vi "Auto_calibrate.vi"(3 "Mode":T4, 5 "Traverse line":T5 {"Row Duration (mins)" format="%#.1f"; "Row No" min=0; "Trace Gas Concentration (%)" min=0.0 format="%#.2f"; "Emission Rate (l/min)" format="%#.2f"; "Tunnel Speed" format="%#.2f"; "Start X" format="%#.2f"; "Start Y" format="%#.2f"; "Start Z" format="%#.2f"; "End X" format="%#.2f"; "End Y" format="%#.2f"; "End Z" format="%#.2f"; "Averaging time (min)" min=0.0 format="%#.1f"}) -> (0 "Error Messages":string, 1 "Status":T2, 2 "Traverse Out":T5 {"Row Duration (mins)" format="%#.1f"; "Row No" min=0; "Trace Gas Concentration (%)" min=0.0 format="%#.2f"; "Emission Rate (l/min)" format="%#.2f"; "Tunnel Speed" format="%#.2f"; "Start X" format="%#.2f"; "Start Y" format="%#.2f"; "Start Z" format="%#.2f"; "End X" format="%#.2f"; "End Y" format="%#.2f"; "End Z" format="%#.2f"; "Averaging time (min)" min=0.0 format="%#.1f"})   [LabVIEW 2010]
uses:
  Gen Trav/Traverse_cluster.ctl
  Gen Trav/Spacing.ctl
  Controls/Multi_run_mode.ctl
  Controls/User_Specific_mode.ctl
  Controls/Auto_Calib_Type.ctl
  Gen Trav/Multi_Run_Status.ctl
  Controls/Auto_Calib_Case.ctl
  Calibration/Calib_mode.ctl
  Controls/Save_Data.ctl
  Controls/Post_Process.ctl
  Controls/Setup.ctl
  Controls/App_Global.ctl
  Globals/Constants_global.vi
  Globals/Meas_global.vi
  Globals/Calib_global.vi
  Globals/Trav_pos_global.vi
  Globals/Plug_in_data_global.vi
  Globals/Extra_Commands_Global.vi
  <vilib>/Analysis/NI_AALBase.lvlib
panel:
  out "Minimum St Dev":dbl[](array[numeric])
  out "Time FFID valve moved":dbl
  out "Wait factor":dbl
  out "Establishment time":string
  out "Orig Calib file string":string
  out "Concentrations":dbl[](array[numeric])
  out "FFID St Dev":dbl[][](array[numeric]) format="%.2f"
  in  "Clear Calib History":bool
  out "Coefficients":dbl[][](array[numeric]) format="%.2f"
  out "Currently in Case":T1
  out "Valve position":dbl format="%.2f"
  out "Currently On":i32
  out "Values":dbl[][](array[numeric]) format="%.2f"
  out "FF Indexes":i16[](array[numeric])
  out "Ch No's":i16[](array[numeric])
  out "No of Calib Points":i32
  out "Root Name":string[](array[string])
  out "Original Calib File":path
  out "Calibration varying":T3
  in  "stop":bool
  out "New Calib Filenames":path[](array[path])
  # "Specific Argument Options\n      Tunnel Speed;1;2;3;4\nOR  Traverse Position\nOR   Concentration"
  # "X           Y            Z"
  # "Start"
  # "End"
  # "X           Y            Z"
  # "Start"
  # "End"
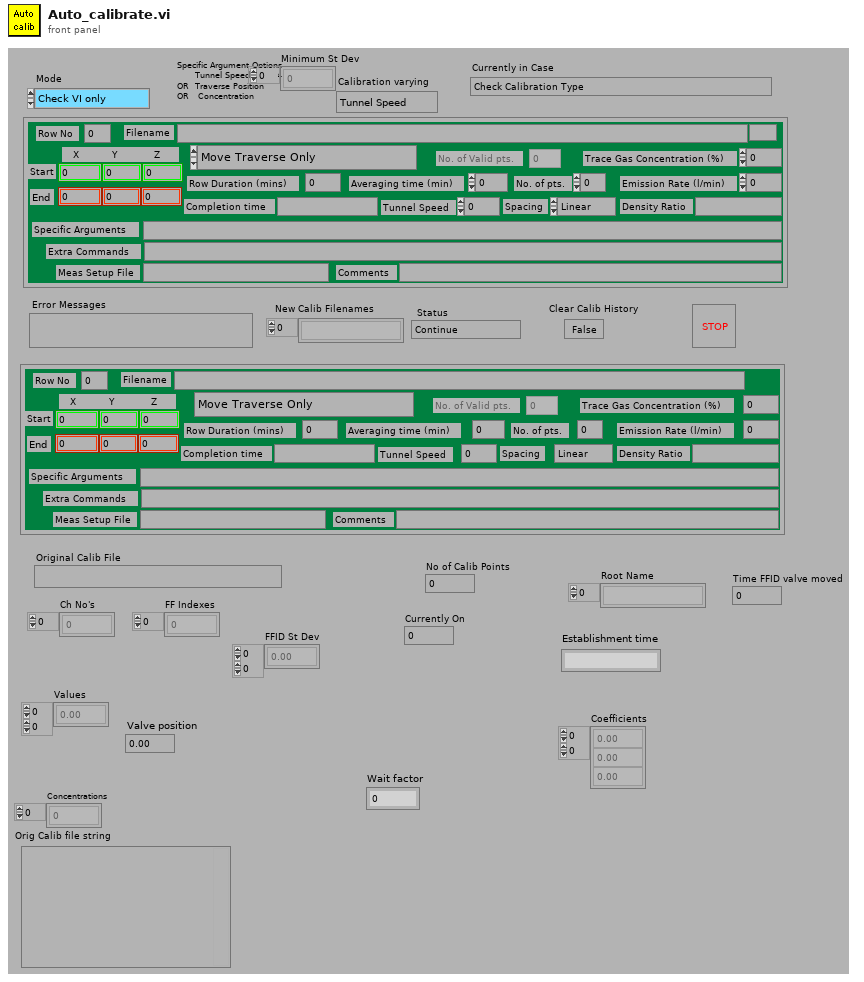
[diagram p1: front panel]
types:
  T1 = typedef "Auto_Calib_Case.ctl" = enum16{"Check Calibration Type", "Check if Original Calib file is Valid", "Get sampling rate etc. from meas setup file", "Setup Calibration Program", "Get Channel Numbers", "Check use latest selected on Mesurement setup files", "Create New Calib Filenames", "Setup Calibration Values in 2D array", "Create Measurement Setup File (Concentration Only)", "Are There Enough Calibration Points", "Set Measurement Conditions", "Measure Calibration Point", "Do Another Calibration Point?", "Skip Next Frame?", "Insert New calibration Filenames into Measurement Setup file", "Warn if FFID calibration is very non linear", "Warn if FFID variance is high", "Insert Bkgnd Variance into calib file", "Warn if FFID voltages are too low", "Warn if Current Calibration fit is poor", "Warn if Calibration Coefficients have significantly altered", "End"}
  T2 = typedef "Multi_Run_Status.ctl" = enum16{"Continue", "Jump to Next Point", "Jump to Next Row", "Jump To Fall Back", "Terminate Run"}
  T3 = typedef "Auto_Calib_Type.ctl" = enum16{"Tunnel Speed", "Traverse Position", "Concentration"}
  T4 = typedef "User_Specific_mode.ctl" = enum16{"Check VI only", "Run VI"}
  T5 = typedef "Traverse_cluster.ctl" = cluster{"Start X":dbl, "Start Y":dbl, "Start Z":dbl, "End X":dbl, "End Y":dbl, "End Z":dbl, "No. of pts.":i32, "Spacing":T6, "Filename":path, "Tunnel Speed":dbl, "Averaging time (min)":dbl, "Extra Commands":string, "Specific Arguments":string, "Emission Rate (l/min)":dbl, "Trace Gas Concentration (%)":dbl, "Density Ratio":string, "Comments":string, "Row No":i32, "Row Type Selector":T7, "Completion time":string, "Row Duration (mins)":dbl, "No. of Valid pts.":i32, "Meas Setup File":string}
  T6 = typedef "Spacing.ctl" = enum16{"Linear", "Log", "Gauss", "Specified", "N/A"}
  T7 = typedef "Multi_run_mode.ctl" = enum16{"Move Traverse Only", "Set Tunnel Speed Only", "Set Source Only", "Set Measurement Conditions", "Single Measurement", "Vertical Profile", "Lateral Profile", "Longitudinal Profile", "Explore Volume", "Multi-Axis Profile", "Auto Calibrate", "Meas Fast FID Bkgnd", "Check Beam Power", "Scanning Valve Measurement", "Run VI Named:", "Set ADAM Ch", "Wait (minutes)", "Send Message", "Synchronize With:", "Fall Back to this Row", "Turn Off Row Repeating", "Blank Row"}
  T8 = typedef "Calib_mode.ctl" = enum16{"Show Setup", "Take a New Calibration Point", "Refit Curve", "Setup Front Panel"}
  T9 = typedef "Save_Data.ctl" = enum16{"Save No Data", "Save Data"}
  T10 = typedef "Post_Process.ctl" = enum16{"Take New Data", "Post Process Raw Data File"}
  T11 = typedef "Setup.ctl" = enum16{"Run Program", "Show Setup", "Save Current Setup", "Setup Front Panel"}
  T12 = typedef "App_Global.ctl" = enum16{"Read Global", "Write to Global", "Initialise Array"}
  T13 = typedef "Cal_Inst_type.ctl" = enum16{"Propeller anemometer", "Pressure Transducer", "Hot wire", "Cross wire velocity", "Cross wire angle", "Generic Linear", "Generic Polynomial", "Generic BackPoly", "Fast FID", "Thermocouple", "Cold wire", "Pulsed Wire"}
  T14 = typedef "Ref_Inst_type.ctl" = enum16{"Propellor anemometer", "Pressure Transducer", "Raw voltage", "Pitot-static tube", "Preston tube", "Generic Linear", "Generic Polynomial", "Thermocouple", "LDA", "Enter Value", "ADAM Channel"}
  T15 = cluster{"2nd Ref type":T14, "2nd inst present":bool}
  T16 = cluster{"high limit (10V)":sgl, "low limit (-10V)":sgl, "Ch No":i16, "Var name":string}[]
  T17 = cluster{"high limit (10V)":sgl, "low limit (-10V)":sgl, "Ch No":i16, "Var name":string}
  T18 = typedef "Inst_type.ctl" = enum16{"Propeller anemometer", "Raw voltage", "Pressure Transducer", "Pitot-static tube", "Preston tube", "Hot wire", "Cross wire 1", "Cross wire 2", "Generic Linear", "Generic Polynomial", "Generic BackPoly", "Fast FID", "Thermocouple", "Cold wire", "Pulsed Wire", "LDA Vel", "LDA Tran time", "LDA Arr time"}
  T19 = cluster{"high limit (10V)":sgl, "low limit (-10V)":sgl, "Ch No":i16, "Calib filename":path, "Inst type":T18, "Symbol":string, "Move channel":bool, "Use Latest":bool, "D":dbl, "Ch Name":string}[]
  T20 = typedef "Status_Cluster.ctl" = cluster{"Status":T2, "Error Type":string, "Error Description":string}
  T21 = typedef "Valco_valve_ph.ctl" = u16
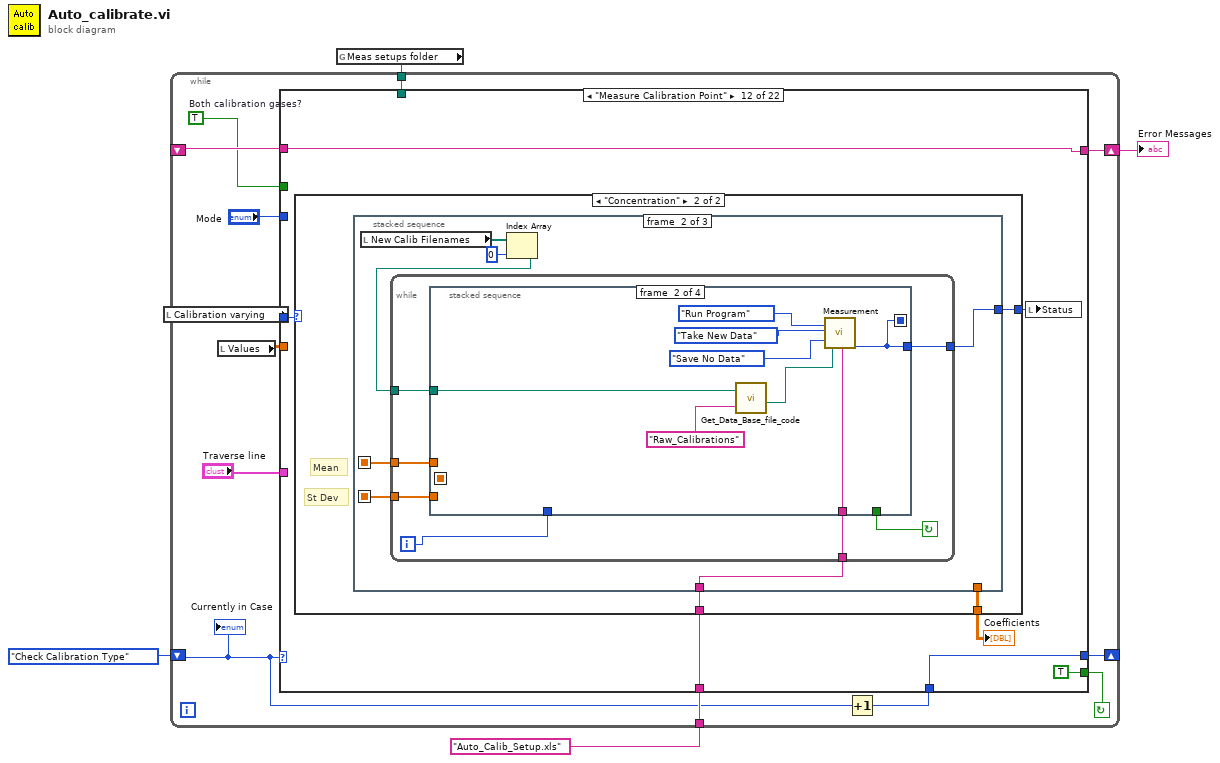
[diagram p0: block diagram]
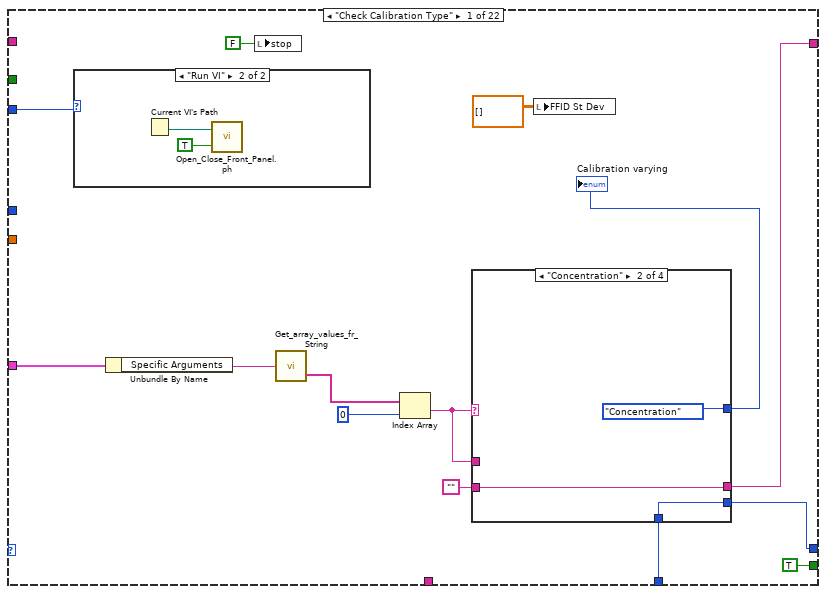
[diagram p2: hidden frame]
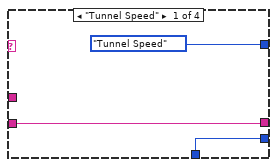
[diagram p4: hidden frame]
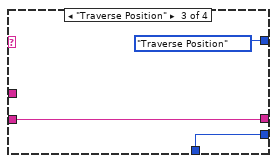
[diagram p5: hidden frame]
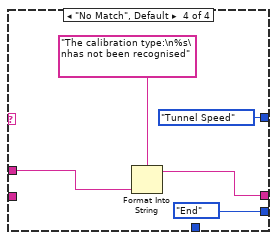
[diagram p6: hidden frame]
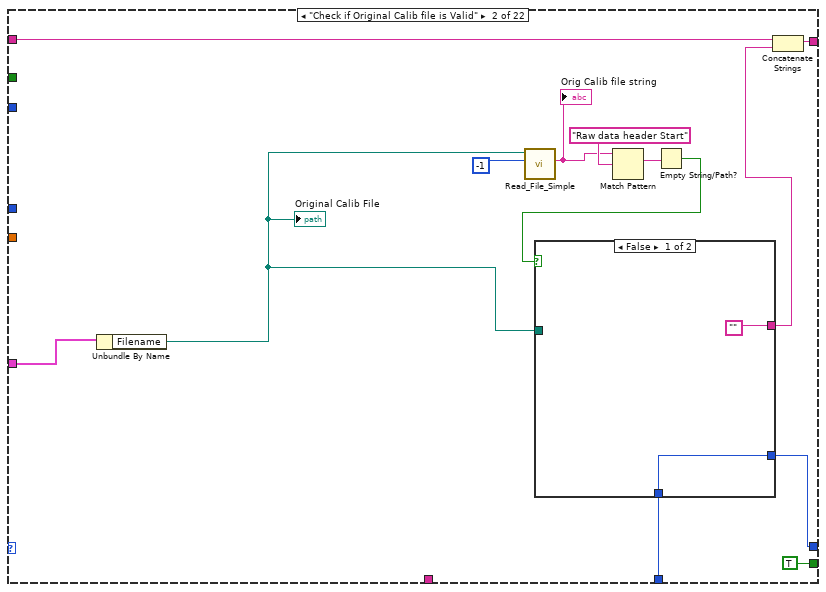
[diagram p7: hidden frame]
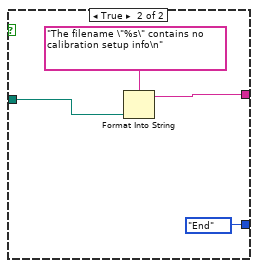
[diagram p8: hidden frame]
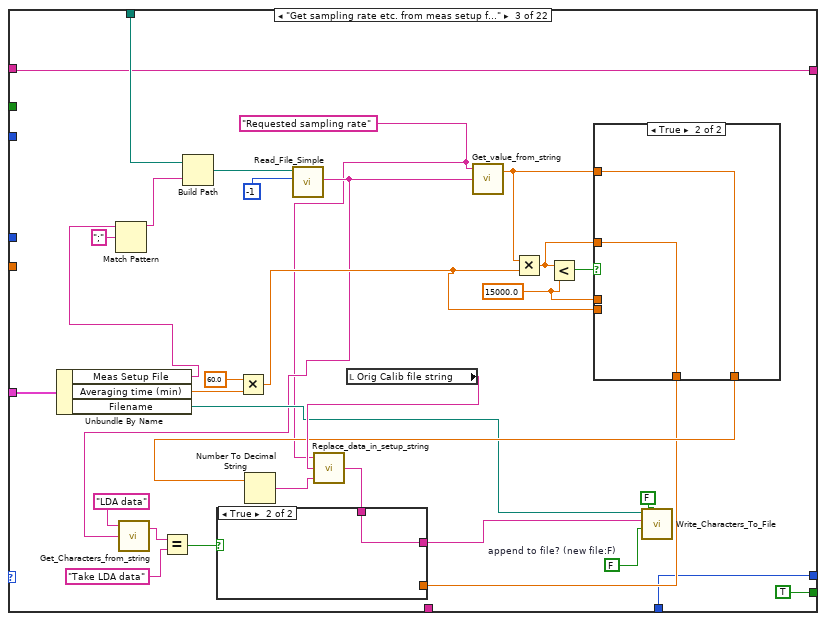
[diagram p9: hidden frame]
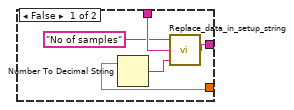
[diagram p10: hidden frame]
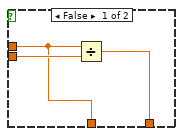
[diagram p11: hidden frame]
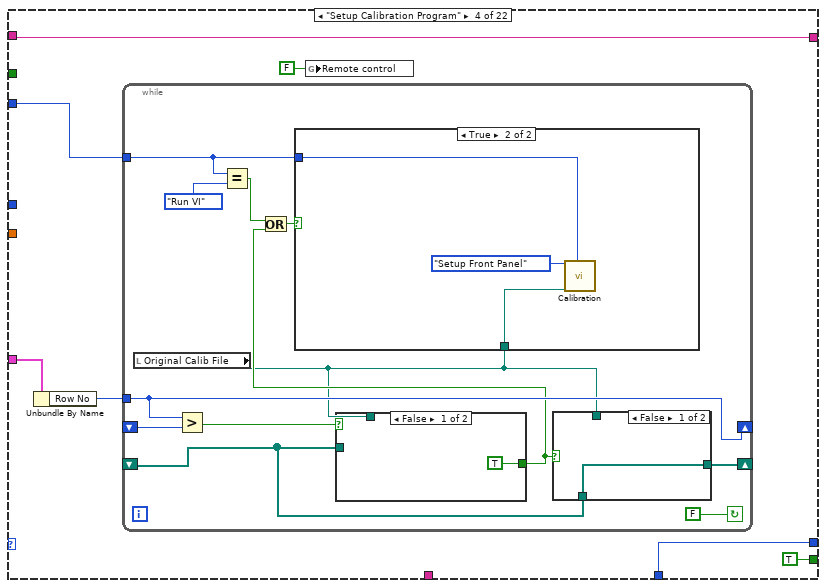
[diagram p12: hidden frame]
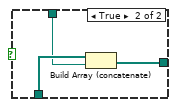
[diagram p13: hidden frame]
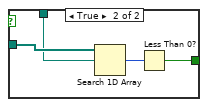
[diagram p15: hidden frame]
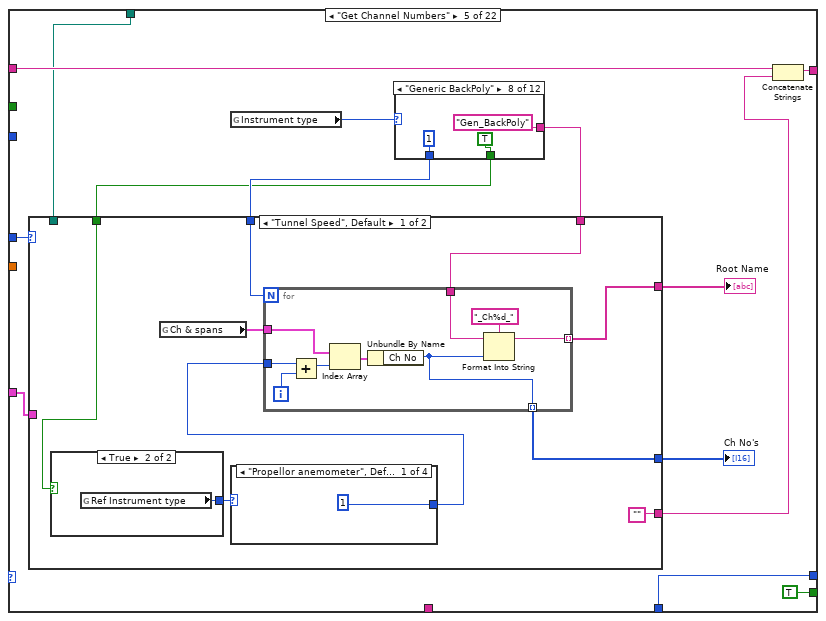
[diagram p16: hidden frame]
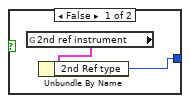
[diagram p17: hidden frame]
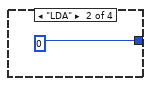
[diagram p18: hidden frame]
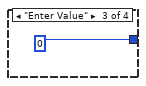
[diagram p19: hidden frame]
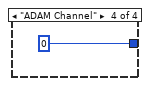
[diagram p20: hidden frame]
diagram:
  n1 = global read "Constants_global.vi" "Meas setups folder"() -> (w1:path)
  n2 = while {
    shift-left: _ -> [w9]
    shift-right: [w10] -> w3
    shift-left: Auto_Calib_Case."Check Calibration Type" ("Currently in Case") -> [w8]
    shift-right: [w7] -> _
    tunnel: "Auto_Calib_Setup.xls" -> [w17]
    tunnel: w1 -> [w5]
    stop <- w13 continue-if-true
    w6 = TRUE  # Both calibration gases?
    n3 = local read "Calibration varying"() -> (w12:T3)
    n4 = local read "Values"() -> (w11:dbl[][])
    n5 = Increment(x=w8) -> (x+1=w14:T1)
    n6 = case shown="\"Measure Calibration Point\"" w8 {
      tunnel: "Traverse line" -> [w31 w60 w98 w112 w143 _ _ w367 w400 _ w577 _ _ _ _ _ _ _ _ _ w993 w1024]
      tunnel: "Mode" -> [w22 _ _ w113 _ _ w318 _ w401 _ w572 _ w737 _ _ _ _ _ _ _ _ w1025]
      tunnel: w17 -> [_ _ _ _ _ _ _ _ w405 _ _ w649 _ _ _ _ _ _ _ _ _ _]
      tunnel: [w20 w50 w78 w115 w146 w264 w315 w358 w403 w540 w565 w648 w738 w764 w774 w795 w833 w898 w916 w972 w1016 w1030] -> w7
      tunnel: w14 -> [w21 w49 w78 w115 w146 w264 w315 w359 w403 w539 w559 w648 _ w763 w773 w795 w833 w898 w916 w972 w1016 w1030]
      tunnel: [TRUE TRUE TRUE TRUE TRUE TRUE TRUE TRUE w399 TRUE TRUE TRUE TRUE TRUE TRUE TRUE TRUE TRUE TRUE TRUE TRUE FALSE] -> w13
      tunnel: w12 -> [_ _ _ _ w150 _ w314 w365 _ _ w563 w650 w736 w762 w776 _ _ _ _ _ _ w1026]
      tunnel: w11 -> [_ _ _ _ _ _ _ _ w398 w549 w576 _ _ _ _ _ w840 _ w922 _ _ _]
      tunnel: [w24 w52 w76 w116 w147 w265 w329 w362 w404 w543 w560 w646 w735 w767 w780 w804 w847 w894 w923 w961 w1009 w1029] -> w10
      tunnel: w9 -> [_ w54 w76 w116 w149 w265 w329 w361 w404 w544 w560 w646 w735 w767 w780 w804 w847 w894 w923 w961 w1009 w1029]
      tunnel: w6 -> [_ _ _ _ _ _ _ w360 _ _ _ _ _ _ _ _ _ _ _ _ _ w1023]
      tunnel: w5 -> [_ _ w97 _ w142 w267 _ _ w402 _ _ _ _ _ _ _ _ _ _ _ _ _]
      frame "Check Calibration Type" {
        n7 = case shown="\"Run VI\"" w22 {
          frame "Check VI only" {
          }
          frame "Run VI" {
            n8 = Current VI's Path() -> (path=w32:path)
            n9 = call "Open_Close_Front_Panel.ph.vi"("Front Panel Window:Open"=TRUE, "VI path"=w32) -> ()  [unwired: 2 out]
          }
        }
        n10 = Unbundle By Name(w31) -> ("Specific Arguments"=w30:string)
        n11 = local write "stop"(FALSE) -> ()
        n12 = call "Get_array_values_fr_String.vi"("String Value"=w30) -> ("String array"=w29:string[])  [unwired: 1 out]
        n13 = Index Array(array=w29, index=0 ("Index")) -> (element=w27:string)
        n14 = case shown="\"Concentration\"" w27 {
          tunnel: [Auto_Calib_Type."Tunnel Speed" ("Calibration varying") Auto_Calib_Type."Concentration" ("Calibration varying") Auto_Calib_Type."Traverse Position" ("Calibration varying") Auto_Calib_Type."Tunnel Speed" ("Calibration varying")] -> w25
          tunnel: w27 -> [_ _ _ w46]
          tunnel: [w35 w38 w41 w44] -> w24
          tunnel: "" -> [w35 w38 w41 _]
          tunnel: w21 -> [w34 w37 w40 _]
          tunnel: [w34 w37 w40 Auto_Calib_Case."End" ("Currently in Case")] -> w20
          frame "Tunnel Speed" {
          }
          frame "Concentration" {
            (unwired) ""
          }
          frame "Traverse Position" {
          }
          frame "No Match", Default {
            n15 = Format Into String(format string="The calibration type:\n%s\nhas not been recognised" ("Format String"), w46) -> (resulting string=w44:string)  [unwired: 2 in, 1 out]
          }
        }
        "Calibration varying" <- w25
        n16 = local write "FFID St Dev"(dbl[][] [] ("FFID Variance")) -> ()
      }
      frame "Check if Original Calib file is Valid" {
        n17 = Unbundle By Name(w60) -> ("Filename"=w48:path)
        "Original Calib File" <- w48
        n18 = call "Read_File_Simple.vi"("Filename"=w48, "number of characters (all:-1)"=-1) -> ("string"=w57:string)  [unwired: 1 in, 7 out]
        "Orig Calib file string" <- w57
        n19 = Match Pattern(string=w57, regular expression="Raw data header Start") -> (match substring=w56:string)  [unwired: 4 out]
        n20 = Empty String/Path?(string/path=w56) -> (empty?=w55:bool)
        n21 = case shown="False" w55 {
          tunnel: w48 -> [_ w66]
          tunnel: ["" w64] -> w53
          tunnel: [w61 Auto_Calib_Case."End" ("Currently in Case")] -> w50
          tunnel: w49 -> [w61 _]
          frame False {
          }
          frame True {
            n22 = Format Into String(format string="The filename \"%s\" contains no calibration setup info\n" ("Format String"), w66) -> (resulting string=w64:string)  [unwired: 2 in, 1 out]
          }
        }
        n23 = Concatenate Strings(w54, w53) -> (w52:string)
      }
      frame "Get sampling rate etc. from meas setup file" {
        w79 = FALSE  # append to file? (new file:F)
        w67 = "Requested sampling rate"
        w86 = 15000.0 ("y")
        n24 = Unbundle By Name(w98) -> ("Meas Setup File"=w74:string, "Averaging time (min)"=w94:dbl, "Filename"=w81:path)
        n25 = Match Pattern(string=w74, regular expression=";") -> (before substring=w73:string)  [unwired: 4 out]
        n26 = Build Path(base path=w97, name or relative path=w73) -> (appended path=w95:path)
        n27 = Multiply(x=60.0, y=w94) -> (x*y=w85:dbl)
        n28 = call "Read_File_Simple.vi"("Filename"=w95, "number of characters (all:-1)"=-1) -> ("string"=w72:string)  [unwired: 1 in, 7 out]
        n29 = call "Get_Characters_from_string.vi"("Input string"=w72, "Variable name"="LDA data") -> ("Value"=w70:string)  [unwired: 1 in, 1 out]
        n30 = Equal?(x=w70, y="Take LDA data") -> (x = y?=w68:bool)
        n31 = local read "Orig Calib file string"() -> (w90:string)
        n32 = call "Get_value_from_string.vi"("Input string"=w72, "Variable name"=w67) -> ("Value"=w89:dbl)  [unwired: 1 in, 1 out]
        n33 = Multiply(x=w89, y=w85) -> (x*y=w84:dbl)
        n34 = Less?(x=w84, y=w86) -> (x < y?=w92:bool)
        n35 = case shown="True" w92 {
          tunnel: w89 -> [_ w109]
          tunnel: [w106 w109] -> w88
          tunnel: w86 -> [w105 _]
          tunnel: w85 -> [w107 _]
          tunnel: [w105 w108] -> w82
          tunnel: w84 -> [_ w108]
          frame False {
            n36 = Divide(x=w105, y=w107) -> (x/y=w106:dbl)
          }
          frame True {
          }
        }
        n37 = Number To Decimal String(number=w88) -> (decimal integer string=w87:string)  [unwired: 1 out]
        n38 = call "Replace_data_in_setup_string.vi"("New data string"=w87, "Input string"=w90, "Variable name"=w67) -> ("Appended string"=w83:string)
        n39 = case shown="True" w68 {
          tunnel: w83 -> [w103 w104]
          tunnel: w82 -> [w100 _]
          tunnel: [w99 w104] -> w80
          frame False {
            n40 = Number To Decimal String(number=w100) -> (decimal integer string=w101:string)  [unwired: 1 out]
            n41 = call "Replace_data_in_setup_string.vi"("New data string"=w101, "Input string"=w103, "Variable name"="No of samples") -> ("Appended string"=w99:string)
          }
          frame True {
          }
        }
        n42 = call "Write_Characters_To_File.vi"("file path (dialog if empty)"=w81, "advisory dialog? (display:T)"=FALSE, "character string"=w80, "append to file? (new file:F)"=w79) -> ()  [unwired: 1 in, 4 out]
      }
      frame "Setup Calibration Program" {
        n43 = Unbundle By Name(w112) -> ("Row No"=w111:i32)
        n44 = while {
          shift-left: _ -> [w120]
          shift-right: [w118] -> _
          tunnel: w111 -> [w127]
          shift-left: _ -> [w128]
          shift-right: [w127] -> _
          tunnel: w113 -> [w125]
          stop <- FALSE continue-if-true
          n45 = local read "Original Calib File"() -> (w119:path)
          n46 = Greater?(x=w127, y=w128) -> (0:w126:bool)
          n47 = Equal?(x=w125, y=User_Specific_mode."Run VI" ("Mode")) -> (x = y?=w123:bool)
          n48 = case shown="False" w126 {
            tunnel: w120 -> [_ w140]
            tunnel: w119 -> [_ w139]
            tunnel: [TRUE w137] -> w121
            frame False {
            }
            frame True {
              n49 = Search 1D Array(1D array=w140, element=w139) -> (index of element=w138:i32)  [unwired: 1 out]
              n50 = Less Than 0?(x=w138) -> (x < 0?=w137:bool)
            }
          }
          n51 = Or(x=w123, y=w121) -> (x .or. y?=w122:bool)
          n52 = case shown="True" w122 {
            tunnel: w125 -> [_ w135]
            tunnel: w119 -> [_ w134]
            frame False {
            }
            frame True {
              n53 = call "Calibration.vi"("Mode"=Calib_mode."Setup Front Panel", "Calib file"=w134, "Simulate/Run"=w135) -> ()  [unwired: 17 out]
            }
          }
          n54 = case shown="False" w121 {
            tunnel: w120 -> [w129 w132]
            tunnel: w119 -> [_ w131]
            tunnel: [w129 w130] -> w118
            frame False {
            }
            frame True {
              n55 = Build Array (concatenate)(w132, w131) -> (w130:path[])
            }
          }
        }
        n56 = global write "Meas_global.vi" "Remote control"(FALSE ("Remote control")) -> ()
      }
      frame "Get Channel Numbers" {
        n57 = global read "Calib_global.vi" "Instrument type"() -> (w154:T13)
        n58 = case shown="\"Generic BackPoly\"" w154 {
          tunnel: ["Prop" "Mano" "HW" "XW" "XW" "Gen_Lin" "Gen_Poly" "Gen_BackPoly" "FF" "Therm" "CW" "PWA"] -> w153
          tunnel: [1 1 1 2 2 1 1 1 1 1 1 1] -> w144
          tunnel: [TRUE TRUE TRUE TRUE FALSE TRUE TRUE TRUE TRUE TRUE TRUE TRUE] -> w141
          frame "Propeller anemometer" {
          }
          frame "Pressure Transducer" {
          }
          frame "Hot wire" {
          }
          frame "Cross wire velocity" {
          }
          frame "Cross wire angle" {
          }
          frame "Generic Linear" {
          }
          frame "Generic Polynomial" {
          }
          frame "Generic BackPoly" {
          }
          frame "Fast FID" {
          }
          frame "Thermocouple" {
          }
          frame "Cold wire" {
          }
          frame "Pulsed Wire" {
          }
        }
        n59 = case shown="\"Tunnel Speed\", Default" w150 {
          tunnel: w153 -> [w161 w197]
          tunnel: [w157 w196] -> w152
          tunnel: [w158 w194] -> w151
          tunnel: ["" w187] -> w148
          tunnel: w144 -> [w159 _]
          tunnel: w143 -> [_ w186]
          tunnel: w142 -> [_ w185]
          tunnel: w141 -> [w155 _]
          frame "Tunnel Speed", Default {
            n60 = case shown="True" w155 {
              tunnel: [w164 w166] -> w163
              frame False {
                n61 = global read "Calib_global.vi" "2nd ref instrument"() -> (w165:T15)
                n62 = Unbundle By Name(w165) -> ("2nd Ref type"=w164:T14)
              }
              frame True {
                n63 = global read "Calib_global.vi" "Ref Instrument type"() -> (w166:T14)
              }
            }
            n64 = global read "Calib_global.vi" "Ch & spans"() -> (w160:T16)
            n65 = case shown="\"Propellor anemometer\", Default" w163 {
              tunnel: [1 i16 0 0 0] -> w156
              frame "Propellor anemometer", Default {
              }
              frame "LDA" {
              }
              frame "Enter Value" {
              }
              frame "ADAM Channel" {
              }
            }
            n66 = for {
              N: w159 -> [_]
              tunnel: [w173] -> w158 mode=indexing
              tunnel: w161 -> [w172]
              tunnel: w160 -> [w171]
              tunnel: [w170] -> w157 mode=indexing
              tunnel: w156 -> [w168]
              i -> [w169]
              n67 = Add(x=w168, y=w169) -> (x+y=w167:i32)
              n68 = Index Array(array=w171, index=w167) -> (element=w175:T17)
              n69 = Unbundle By Name(w175) -> ("Ch No"=w173:i16)
              n70 = Format Into String(format string="_Ch%d_" ("Format String"), initial string=w172, w173) -> (resulting string=w170:string)  [unwired: 1 in, 1 out]
            }
          }
          frame "Concentration" {
            w193 = i16[] []
            n71 = Unbundle By Name(w186) -> ("Meas Setup File"=w181:string)
            n72 = Match Pattern(string=w181, regular expression=";") -> (before substring=w180:string)  [unwired: 4 out]
            n73 = Build Path(base path=w185, name or relative path=w180) -> (appended path=w184:path)
            n74 = call "Read_raw_inst_setup.vi"("Setup file"=w184) -> ("Ch & spans choices"=w183:T19)  [unwired: 18 out]
            n75 = for {
              tunnel: w183 -> [w208] mode=indexing
              tunnel: w197 -> [w207]
              shift-right: [w203] -> w196
              shift-left: string[] [] -> [w204]
              shift-right: [w201] -> w194
              shift-left: w193 -> [w202]
              shift-right: [w200] -> w192
              shift-left: w193 -> [w199]
              i -> [w198]
              n76 = Unbundle By Name(w208) -> ("Ch No"=w206:i16, "Inst type"=w205:T18)
              n77 = case shown="\"Fast FID\"" w205 {
                tunnel: w207 -> [_ w213]
                tunnel: w206 -> [_ w215]
                tunnel: w204 -> [w211 w223]
                tunnel: [w211 w222] -> w203
                tunnel: w202 -> [w210 w221]
                tunnel: [w210 w220] -> w201
                tunnel: w199 -> [w209 w218]
                tunnel: [w209 w219] -> w200
                tunnel: w198 -> [_ w217]
                frame "Generic Linear", Default {
                }
                frame "Fast FID" {
                  n78 = To Word Integer(number=w217) -> (16bit integer=w216:i16)
                  n79 = Format Into String(format string="_Ch%d_", initial string=w213, w215) -> (resulting string=w212:string)  [unwired: 1 in, 1 out]
                  n80 = Build Array (concatenate)(w221, w215) -> (w220:i16[])
                  n81 = Build Array (concatenate)(w218, w216) -> (w219:i16[])
                  n82 = Build Array (concatenate)(w223, w212) -> (w222:string[])
                }
              }
            }
            "FF Indexes" <- w192
            n83 = Array Size(array=w192) -> (size(s)=w191:i32)
            n84 = Greater Than 0?(x=w191) -> (x > 0?=w190:bool)
            n85 = Select(t="", s=w190, f="There are no Fast Fid channels selected on the current setup of the measurement program.") -> (s? t:f=w187:string)
          }
        }
        "Root Name" <- w152
        "Ch No's" <- w151
        n86 = Concatenate Strings(w149, w148) -> (w147:string)
      }
      frame "Check use latest selected on Mesurement setup files" {
        n87 = global read "Trav_pos_global.vi" "Measurement setup files"() -> (w260:string[])
        n88 = local read "Ch No's"() -> (w266:i16[])
        n89 = Build Array (concatenate)(w260, "Current_Setup.xls") -> (w261:string[])
        n90 = for {
          tunnel: w267 -> [w270]
          tunnel: w261 -> [w269] mode=indexing
          tunnel: w266 -> [w268]
          n91 = stacked-sequence {
            seq-local: [w271 _ _] -> [_ w277 w305]
            seq-local: [_ w275 _] -> [_ _ w303]
            tunnel: w270 -> [w274 _ w302]
            tunnel: w269 -> [w273 _ w301]
            tunnel: w268 -> [_ w276 _]
            frame #0 {
              n92 = Build Path(base path=w274, name or relative path=w273) -> (appended path=w272:path)
              n93 = call "Read_File_Simple.vi"("Filename"=w272) -> ("string"=w271:string)  [unwired: 2 in, 7 out]
            }
            frame #1 {
              n94 = while {
                shift-right: [w282] -> w275
                shift-left: w277 -> [w283]
                tunnel: w276 -> [w286]
                i -> [w290]
                stop <- w279 continue-if-true
                n95 = Increment(x=w290) -> (x+1=w284:i32)
                n96 = Format Into String(format string="An ch %d Ch No", w284) -> (resulting string=w289:string)  [unwired: 2 in, 1 out]
                n97 = call "Get_value_from_string.vi"("Input string"=w283, "Variable name"=w289) -> ("Status"=w288:enum16{"Char in string", "Char not in string"}, "Value"=w287:dbl)  [unwired: 1 in]
                n98 = To Long Integer(number=w287) -> (32bit integer=w285:i32)
                n99 = Search 1D Array(1D array=w286, element=w285) -> (index of element=w281:i32)  [unwired: 1 in]
                n100 = Greater Or Equal To 0?(x=w281) -> (x >= 0?=w280:bool)
                n101 = case shown="\"Char in string\"" w288 {
                  tunnel: [TRUE FALSE] -> w279
                  frame "Char in string" {
                  }
                  frame "Char not in string" {
                  }
                }
                n102 = And(x=w280, y=w279) -> (x .and. y?=w278:bool)
                n103 = case shown="True" w278 {
                  tunnel: w284 -> [w294 _]
                  tunnel: w283 -> [w293 w298]
                  tunnel: [w292 w298] -> w282
                  frame True {
                    n104 = Format Into String(format string="An ch %d Use latest Calib", w294) -> (resulting string=w296:string)  [unwired: 2 in, 1 out]
                    n105 = call "Replace_data_in_setup_string.vi"("New data string"="TRUE" ("Replace with"), "Input string"=w293, "Variable name"=w296) -> ("Appended string"=w292:string)
                  }
                  frame False {
                  }
                }
              }
            }
            frame #2 {
              n106 = Equal?(x=w305, y=w303) -> (x = y?=w304:bool)
              n107 = case shown="True" w304 {
                tunnel: w302 -> [w308 _]
                tunnel: w303 -> [w311 _]
                tunnel: w301 -> [w307 _]
                frame False {
                  w310 = FALSE  # append to file? (new file:F)
                  n108 = Build Path(base path=w308, name or relative path=w307) -> (appended path=w306:path)
                  n109 = call "Write_Characters_To_File.vi"("file path (dialog if empty)"=w306, "advisory dialog? (display:T)"=FALSE, "character string"=w311, "append to file? (new file:F)"=w310) -> ()  [unwired: 1 in, 4 out]
                }
                frame True {
                }
              }
            }
          }
        }
      }
      frame "Create New Calib Filenames" {
        n110 = local read "Original Calib File"() -> (w327:path)
        n111 = Get Date/Time String(date format (0)=enum16{"short", "long", "abbreviated"}."short") -> (date string=w322:string)  [unwired: 3 out]
        n112 = Strip Path(path=w327) -> (stripped path=w317:path)  [unwired: 1 out]
        n113 = local read "Root Name"() -> (w313:string[])
        n114 = case shown="\"Tunnel Speed\", Default" w314 {
          tunnel: w313 -> [_ w334]
          tunnel: [1 w333] -> w312
          frame "Tunnel Speed", Default {
          }
          frame "Concentration" {
            n115 = Array Size(array=w334) -> (size(s)=w333:i32)
          }
        }
        n116 = call "Replace_Character.vi"("Replace with"="-", "Input String"=w322, "Search For"="/") -> ("Output string"=w319:string)  [unwired: 1 out]
        n117 = List Folder(path=w317) -> (filenames=w331:string[])  [unwired: 1 in, 5 out]
        n118 = To Upper Case(1:w331) -> (0:w330:string[])
        n119 = for {
          N: w312 -> [_]
          tunnel: w313 -> [w337] mode=indexing
          tunnel: w330 -> [w341]
          tunnel: w317 -> [w340]
          tunnel: [w336] -> w326 mode=indexing
          tunnel: w319 -> [w338]
          tunnel: w318 -> [w335]
          n120 = while {
            tunnel: w337 -> [w348]
            tunnel: w338 -> [w349]
            tunnel: [w344] -> w339
            tunnel: w341 -> [w351]
            i -> [w353]
            stop <- w355 continue-if-true
            n121 = Increment(x=w353) -> (x+1=w350:i32)
            n122 = Format Into String(format string="%s_%d.xls" ("Format String"), initial string=w348, w349, w350) -> (resulting string=w345:string)  [unwired: 1 in, 1 out]
            n123 = call "Replace_Character.vi"("Replace with"="_", "Input String"=w345, "Search For"=" ") -> ("Output string"=w344:string)  [unwired: 1 out]
            n124 = To Upper Case(1:w344) -> (0:w354:string)
            n125 = Search 1D Array(1D array=w351, element=w354) -> (index of element=w356:i32)  [unwired: 1 out]
            n126 = Not Equal?(x=w356, y=-1) -> (x != y?=w355:bool)
          }
          n127 = Build Path(base path=w340, name or relative path=w339) -> (appended path=w336:path)
          n128 = case shown="\"Run VI\"" w335 {
            tunnel: w336 -> [_ w342]
            frame "Check VI only" {
            }
            frame "Run VI" {
              n129 = call "Calibration.vi"("Mode"=Calib_mode."Setup Front Panel", "Calib file"=w342) -> ()  [unwired: 1 in, 17 out]
            }
          }
        }
        "New Calib Filenames" <- w326
        n130 = Index Array(array=w326, index=0 ("Index")) -> (element=w324:path)
        n131 = global write "Meas_global.vi" "Results file"(w324) -> ()
        "Establishment time" <- "!Establish Exp Conditions (s) = 15" ("Message")
      }
      frame "Setup Calibration Values in 2D array" {
        n132 = case shown="\"Concentration\"" w365 {
          tunnel: [w376 w382 w397] -> w364
          tunnel: w367 -> [w371 _ w396]
          tunnel: ["" "" w395] -> w363
          tunnel: w360 -> [_ w380 _]
          tunnel: w359 -> [w370 w379 w394]
          tunnel: [w369 w379 w393] -> w358
          frame "Tunnel Speed" {
            n133 = Unbundle By Name(w371) -> ("Specific Arguments"=w374:string)
            n134 = call "Get_array_values_fr_String.vi"("String Value"=w374) -> ("Numeric Array"=w372:dbl[])  [unwired: 1 out]
            n135 = Array Subset(array=w372, index=1 ("Array Index")) -> (w368:dbl[])  [unwired: 1 in]
            n136 = for {
              tunnel: w368 -> [w378] mode=indexing
              tunnel: [w377] -> w376 mode=indexing
              n137 = Build Array(w378) -> (w377:dbl[])
            }
            n138 = Increment(x=w370) -> (x+1=w369:T1)
          }
          frame "Concentration" {
            n139 = case shown="True" w380 {
              tunnel: [w384 w388] -> w383
              frame True {
                n140 = Build Array(3.0, 2.0, 1.0) -> (w384:dbl[])
              }
              frame False {
                n141 = Build Array(1.0, 3.0) -> (w388:dbl[])
              }
            }
            n142 = for {
              tunnel: w383 -> [w392] mode=indexing
              tunnel: [w391] -> w382 mode=indexing
              n143 = Build Array(w392) -> (w391:dbl[])
            }
          }
          frame "Traverse Position" {
            n144 = call "Create_Pos_array.vi"("Traverse line"=w396) -> ("Error Messages"=w395:string, "Array of Positions"=w397:dbl[][])  [unwired: 5 in, 2 out]
            n145 = Increment(x=w394) -> (x+1=w393:T1)
          }
        }
        "Values" <- w364
        n146 = Concatenate Strings(w361, w363) -> (w362:string)
      }
      frame "Create Measurement Setup File (Concentration Only)" {
        n147 = stacked-sequence {
          seq-local: [w416 _ _ _ _ _ _] -> [_ w435 _ _ _ _ _]
          seq-local: [_ w433 _ _ _ _ _] -> [_ _ w456 _ _ _ _]
          seq-local: [_ _ _ _ w478 _ _] -> [_ _ _ _ _ w491 _]
          seq-local: [_ _ _ _ w483 _ _] -> [_ _ _ _ _ w492 _]
          tunnel: w402 -> [w407 _ w457 _ _ _ _]
          tunnel: w405 -> [_ _ w458 _ _ _ _]
          tunnel: w401 -> [_ _ _ w464 _ w494 w524]
          tunnel: w400 -> [w413 _ _ _ w490 w495 _]
          tunnel: [_ _ _ _ _ w493 _] -> w399
          tunnel: w398 -> [_ _ _ w467 _ _ _]
          frame #0 {
            w420 = TRUE  # Show Dialog?
            n148 = Unbundle By Name(w413) -> ("Meas Setup File"=w414:string)
            n149 = Match Pattern(string=w414, regular expression=";") -> (before substring=w412:string)  [unwired: 4 out]
            n150 = Build Path(base path=w407, name or relative path=w412) -> (appended path=w421:path)
            n151 = Format Into String(format string="Meas Setup File   %s", w407) -> (resulting string=w406:string)  [unwired: 2 in, 1 out]
            n152 = call "Read_spec_No_of_Characters.vi"("Filename"=w421) -> ("character string"=w422:string)  [unwired: 1 out]
            n153 = call "Get_string_subset.vi"("String Name"=w406, "Show Dialog?"=w420, "String to split"=w422, "File Label"="Raw data header") -> ("Output string"=w409:string)  [unwired: 1 out]
            n154 = call "Get_value_from_string.vi"("Input string"=w409, "Variable name"="No of analogue inst") -> ("Value"=w410:dbl)  [unwired: 1 in, 1 out]
            n155 = for {
              N: w410 -> [_]
              shift-right: [w424] -> w419
              shift-left: w409 -> [w426]
              i -> [w430]
              n156 = Increment(x=w430) -> (x+1=w429:i32)
              n157 = Number To Decimal String(number=w429) -> (decimal integer string=w432:string)  [unwired: 1 out]
              n158 = Concatenate Strings("An ch ", w432, " Inst type") -> (w427:string)
              n159 = call "Replace_data_in_setup_string.vi"("New data string"="Raw voltage", "Input string"=w426, "Variable name"=w427) -> ("Appended string"=w424:string)
            }
            n160 = call "Replace_data_in_setup_string.vi"("New data string"="No LDA data", "Input string"=w419, "Variable name"="LDA data" ("Label for characters")) -> ("Appended string"=w416:string)
          }
          frame #1 {
            n161 = global read "Calib_global.vi" "New Setup String"() -> (w436:string)
            n162 = for {
              N: 4 -> [_]
              shift-right: [w441] -> w433
              shift-left: w435 -> [w442]
              tunnel: w436 -> [w438]
              i -> [w440]
              n163 = case shown="3" w440 {
                tunnel: [w445 w448 w451 "No of blocks"] -> w439
                tunnel: w438 -> [w444 w447 w450 _]
                tunnel: [w443 w446 w449 "1" ("Value")] -> w437
                frame 0, Default {
                  w445 = "No of samples"
                  n164 = call "Get_Characters_from_string.vi"("Input string"=w444, "Variable name"=w445) -> ("Value"=w443:string)  [unwired: 1 in, 1 out]
                }
                frame 2 {
                  w448 = "Actual sampling rate"
                  n165 = call "Get_Characters_from_string.vi"("Input string"=w447, "Variable name"=w448) -> ("Value"=w446:string)  [unwired: 1 in, 1 out]
                }
                frame 3 {
                  w451 = "Board type"
                  n166 = call "Get_Characters_from_string.vi"("Input string"=w450, "Variable name"=w451) -> ("Value"=w449:string)  [unwired: 1 in, 1 out]
                }
                frame 1 {
                }
              }
              n167 = call "Replace_data_in_setup_string.vi"("New data string"=w437, "Input string"=w442, "Variable name"=w439) -> ("Appended string"=w441:string)
            }
          }
          frame #2 {
            w462 = FALSE  # advisory dialog? (display:T)
            w463 = FALSE  # append to file? (new file:F)
            n168 = call "Remove_Plug_Ins_etc.vi"("Input String"=w456) -> ("Output string"=w455:string)
            n169 = call "Add_label_to_string.vi"("String to write"=w455, "File Label"="Raw data header") -> ("Output string"=w459:string)
            n170 = Build Path(base path=w457, name or relative path=w458) -> (appended path=w454:path)
            n171 = call "Add_length_to_string.vi"("String in"=w459) -> ("String out"=w461:string)
            n172 = call "Write_Characters_To_File.vi"("file path (dialog if empty)"=w454, "advisory dialog? (display:T)"=w462, "character string"=w461, "append to file? (new file:F)"=w463) -> ()  [unwired: 1 in, 4 out]
          }
          frame #3 {
            w466 = 0 ("Index")
            w471 = 0.0 ("Input Element")
            n173 = Index Array(array=w467, index (row)=w466, index (col)=w466) -> (element=w465:dbl)
            n174 = case shown="\"Run VI\"" w464 {
              tunnel: w465 -> [_ w474]
              frame "Check VI only" {
              }
              frame "Run VI" {
                n175 = flat-sequence {
                  tunnel: w474 -> [w475]
                  frame #0 {
                    n176 = call "Fast_FID_Valve_Control.vi"("Requested Position"=w475) -> ()  [unwired: 7 out]
                  }
                  frame #1 {
                    n177 = Get Date/Time In Seconds() -> (seconds since 1Jan1904=w477:timestamp)
                    n178 = To Double Precision Float(number=w477) -> (double precision float=→"Time FFID valve moved":dbl)
                  }
                }
              }
            }
            n179 = Build Array("GMU:Calibration:Gas 1", "GMU:Calibration:Gas 2") -> (w473:string[])
            n180 = call "Get_Current_Scan_client.vi"("ADAM Ch Names"=w473) -> ("Numerical Values"=w472:dbl[])  [unwired: 3 out]
            n181 = Build Array (concatenate)(w471, w471, w472, w471) -> (→"Concentrations":dbl[])
          }
          frame #4 {
            n182 = Unbundle By Name(w490) -> ("Extra Commands"=w489:string, "Start X"=w487:dbl, "Start Y"=w486:dbl, "Start Z"=w485:dbl)
            n183 = Build Array(w487, w486, w485) -> (w483:dbl[])
            n184 = call "Which_Trav_Setup.vi"("Extra Command String"=w489) -> ("Traverse Setup"=w488:string)
            n185 = call "Read_Traverse_Pos_File.vi"("Traverse Name"=w488) -> ("Tunnel Coordinates"=w484:dbl[])
            n186 = Subtract(x=w484, y=w483) -> (x-y=w482:dbl[])
            n187 = Absolute Value(x=w482) -> (abs(x)=w481:dbl[])
            n188 = Less?(x=w481, y=0.5) -> (x < y?=w479:bool[])
            n189 = And Array Elements(Boolean array=w479) -> (logical AND=w478:bool)
          }
          frame #5 {
            n190 = case shown="False" w491 {
              tunnel: w495 -> [w505 _]
              tunnel: w494 -> [w501 _]
              tunnel: [w497 TRUE] -> w493
              tunnel: w492 -> [w496 _]
              frame False {
                w500 = dbl[] [30.0, 15.0, 0.0] ("appended array")
                n191 = call "Coordinate_Trans_.vi"("Input Position"=w496) -> ("X"=w502:dbl, "Y"=w503:dbl, "Z"=w504:dbl)
                n192 = Array Size(array=w500) -> (size(s)=w499:i32)
                n193 = Decrement(x=w499) -> (x-1=w498:i32)
                n194 = while {
                  tunnel: w501 -> [w514]
                  tunnel: w505 -> [w520]
                  tunnel: w500 -> [w519] mode=indexing
                  tunnel: w504 -> [w517]
                  tunnel: w503 -> [w516]
                  tunnel: w502 -> [w515]
                  tunnel: w498 -> [w510]
                  tunnel: [w506] -> w497
                  i -> [w511]
                  stop <- w507 continue-if-true
                  n195 = Add(x=w517, y=w519) -> (x+y=w518:dbl)
                  n196 = Less?(x=w511, y=w510) -> (x < y?=w508:bool)
                  n197 = Bundle By Name(cluster=w520, "Start X"=w515, "Start Y"=w516, "Start Z"=w518) -> (w521:T5)
                  n198 = call "Set_Traverse_Position.vi"("Simulate/Run"=w514, "Currently on Point"=1, "Traverse line"=w521) -> ("Status Cluster"=w509:T20)  [unwired: 2 out]
                  n199 = Unbundle By Name(w509) -> ("Status"=w512:T2)
                  n200 = call "Prog_Status_Handler.vi"("Status Cluster"=w509, "Simulate/Run"=w514) -> ()  [unwired: 2 out]
                  n201 = local write "Status"(w512) -> ()
                  n202 = Equal?(x=w512, y=Multi_Run_Status."Continue" ("Status")) -> (x = y?=w506:bool)
                  n203 = And(x=w506, y=w508) -> (x .and. y?=w507:bool)
                }
              }
              frame True {
              }
            }
          }
          frame #6 {
            n204 = case shown="\"Run VI\"" w524 {
              frame "Check VI only", Default {
              }
              frame "Run VI" {
                n205 = while {
                  shift-right: [w536] -> _
                  shift-left: _ -> [w537]
                  tunnel: [w535] -> w530
                  stop <- TRUE stop-if-true
                  n206 = Get Date/Time In Seconds() -> (seconds since 1Jan1904=w536:timestamp)
                  n207 = Subtract(x=w536, y=w537) -> (x-y=w535:dbl)
                }
                n208 = Divide(x=w530, y=3600.0) -> (x/y=w529:dbl)
                n209 = Multiply(x=w529, y=0.2) -> (x*y=w527:dbl)
                n210 = Add(x=w527, y=0.8) -> (x+y=w525:dbl)
                n211 = In Range and Coerce(upper limit=2.0, x=w525, lower limit=1.0) -> (coerced(x)=→"Wait factor":dbl)  [unwired: 1 out]
              }
            }
          }
        }
      }
      frame "Are There Enough Calibration Points" {
        n212 = Array Size(array=w549) -> (size(s)=w550:i32[])
        n213 = Index Array(array=w550, index=0 ("Index")) -> (element=w545:i32)
        "No of Calib Points" <- w545
        n214 = Greater?(x=w545, y=1) -> (0:w546:bool)
        n215 = case shown="False" w546 {
          tunnel: ["Less than two calibration points have been specified\n" ""] -> w542
          tunnel: [Auto_Calib_Case."End" ("Currently in Case") w554] -> w540
          tunnel: w539 -> [_ w554]
          frame False {
          }
          frame True {
          }
        }
        n216 = Concatenate Strings(w544, w542) -> (w543:string)
        "Currently On" <- 1 ("Currently On")
      }
      frame "Set Measurement Conditions" {
        n217 = local read "Currently On"() -> (w564:i32)
        n218 = Decrement(x=w564) -> (x-1=w575:i32)
        n219 = Index Array(array=w576, index (row)=w575) -> (element=w574:dbl[])  [unwired: 1 in]
        n220 = case shown="\"Concentration\"" w563 {
          tunnel: w574 -> [w592 w609 w626]
          tunnel: w572 -> [_ _ w624]
          tunnel: w577 -> [w590 w605 w615]
          tunnel: [w591 w604 w613] -> w558
          tunnel: w564 -> [w586 _ w616]
          tunnel: [w589 w603 w620] -> w556
          frame "Tunnel Speed" {
            n221 = Index Array(array=w592, index=0 ("Index")) -> (element=w579:dbl)
            n222 = while {
              shift-right: [w600] -> w581
              shift-left: _ -> [w599]
              tunnel: w579 -> [w602]
              tunnel: [w600] -> w588
              tunnel: [w599] -> w587
              stop <- FALSE continue-if-true
              n223 = Greater Than 0?(x=w602) -> (x > 0?=w600:bool)
            }
            n224 = Exclusive Or(1:w587, 2:w588) -> (0:w584:bool)
            n225 = Greater?(x=w586, y=1) -> (0:w583:bool)
            n226 = And(x=w584, y=w583) -> (x .and. y?=w582:bool)
            n227 = case shown="False" w581 {
              tunnel: [w594 w596] -> w580
              tunnel: w579 -> [w595 w596]
              frame False {
                n228 = Negate(x=w595) -> (-x=w594:dbl)
              }
              frame True {
              }
            }
            n229 = case shown="True" w582 {
              frame False {
              }
              frame True {
                n230 = call "Wait_Seconds_with_display.vi"("Message"="Please rotate the probe you are calibrating", "Seconds to wait"=10000.0) -> ()  [unwired: 2 out]
              }
            }
            n231 = local read "Establishment time"() -> (w589:string)
            n232 = Bundle By Name(cluster=w590, "Tunnel Speed"=w580) -> (w591:T5)
          }
          frame "Traverse Position" {
            n233 = Index Array(array=w609, index=0 ("Index")) -> (element=w608:dbl)
            n234 = Index Array(array=w609, index=1 ("Index")) -> (element=w607:dbl)
            n235 = Index Array(array=w609, index=2 ("Index")) -> (element=w606:dbl)
            n236 = local read "Establishment time"() -> (w603:string)
            n237 = Bundle By Name(cluster=w605, "Start X"=w608, "Start Y"=w607, "Start Z"=w606) -> (w604:T5)
          }
          frame "Concentration" {
            w614 = nan ("Start X")
            n238 = local read "Wait factor"() -> (w619:dbl)
            n239 = Index Array(array=w626, index=0 ("Index")) -> (element=w617:dbl)
            n240 = case shown="3" w616 {
              tunnel: [w628 w636 100.0] -> w618
              tunnel: w619 -> [w634 w637 _]
              frame 1, Default {
                n241 = local read "Time FFID valve moved"() -> (w631:dbl)
                n242 = Get Date/Time In Seconds() -> (seconds since 1Jan1904=w633:timestamp)
                n243 = Multiply(x=w634, y=35.0) -> (x*y=w630:dbl)
                n244 = To Double Precision Float(number=w633) -> (double precision float=w632:dbl)
                n245 = Subtract(x=w632, y=w631) -> (x-y=w629:dbl)
                n246 = Subtract(x=w630, y=w629) -> (x-y=w628:dbl)
              }
              frame 2 {
                n247 = Multiply(x=w637, y=25.0) -> (x*y=w636:dbl)
              }
              frame 3 {
              }
            }
            n248 = case shown="\"Run VI\"" w624 {
              tunnel: w617 -> [w641 w642]
              tunnel: [w640 w643] -> w625
              frame "Check VI only" {
                n249 = To Long Integer(number=w641) -> (32bit integer=w640:i32)
              }
              frame "Run VI" {
                n250 = call "Fast_FID_Valve_Control.vi"("Requested Position"=w642) -> ("Achieved Posn."=w643:T21)  [unwired: 6 out]
              }
            }
            n251 = Number To Decimal String(number=w618) -> (decimal integer string=w621:string)  [unwired: 1 out]
            n252 = Concatenate Strings("!Establish Exp Conditions (s) = " ("Message"), w621) -> (w620:string)
            n253 = To Double Precision Float(number=w625) -> (double precision float=→"Valve position":dbl)
            n254 = Bundle By Name(cluster=w615, "Start X"=w614, "Start Y"=w614, "Start Z"=w614) -> (w613:T5)
          }
        }
        n255 = call "Add_Extra_Command.vi"("Traverse line"=w558, "Extra Command"=w556) -> ("Traverse line Out"=w557:T5)
        n256 = call "Set_Measurement_Conditions.vi"("Simulate/Run"=w572, "Currently on Point"=1, "Traverse line"=w557) -> ("Status Cluster"=w562:T20)  [unwired: 2 out]
        n257 = Unbundle By Name(w562) -> ("Status"=w561:T2)
        "Status" <- w561
        n258 = Equal?(x=w561, y=Multi_Run_Status."Continue" ("Status")) -> (x = y?=w568:bool)
        n259 = Equal?(x=User_Specific_mode."Run VI" ("Mode"), y=w572) -> (x = y?=w569:bool)
        n260 = Increment(x=w559) -> (x+1=w566:T1)
        n261 = And(x=w568, y=w569) -> (x .and. y?=w567:bool)
        n262 = Select(t=w559, s=w567, f=w566) -> (s? t:f=w565:T1)
      }
      frame "Measure Calibration Point" {
        n263 = case shown="\"Concentration\"" w650 {
          tunnel: w649 -> [_ w659]
          tunnel: [w653 w658] -> w645
          tunnel: [w651 w657] -> w644
          frame "Tunnel Speed", Default {
            n264 = local read "New Calib Filenames"() -> (w654:path[])
            n265 = Index Array(array=w654, index=0 ("Index")) -> (element=w655:path)
            n266 = call "Calibration.vi"("Mode"=Calib_mode."Take a New Calibration Point", "Calib file"=w655) -> ("Coefficients"=w651:dbl[][], "Status Out"=w653:T2)  [unwired: 1 in, 15 out]
          }
          frame "Concentration" {
            # "St Dev"
            # "Mean"
            n267 = stacked-sequence {
              seq-local: [_ w663 _] -> [_ _ w707]
              seq-local: [_ w662 _] -> [_ _ w706]
              tunnel: w659 -> [_ w666 _]
              tunnel: [_ w664 _] -> w658
              tunnel: [_ _ w708] -> w657
              frame #0 {
                n268 = global write "Meas_global.vi" "Remote control"(TRUE ("Remote control")) -> ()
                n269 = global write "Meas_global.vi" "Raw data option"(enum16{"Save raw data", "Raw data not saved"}."Save raw data" ("Raw data option")) -> ()
              }
              frame #1 {
                n270 = local read "New Calib Filenames"() -> (w667:path[])
                n271 = Index Array(array=w667, index=0 ("Index")) -> (element=w665:path)
                n272 = while {
                  tunnel: [w675] -> w664
                  tunnel: w665 -> [w674]
                  tunnel: w666 -> [w672]
                  tunnel: [w671] -> w663
                  tunnel: [w670] -> w662
                  i -> [w669]
                  stop <- w673 continue-if-true
                  n273 = stacked-sequence {
                    seq-local: [_ w677 _ _] -> [_ _ _ w700]
                    seq-local: [_ _ w685 _] -> [_ _ _ w704]
                    tunnel: [_ w677 _ _] -> w675
                    tunnel: w674 -> [_ w682 _ _]
                    tunnel: [_ _ _ w695] -> w673
                    tunnel: w672 -> [_ w678 _ _]
                    tunnel: [_ _ w686 _] -> w671
                    tunnel: [_ _ w685 _] -> w670
                    tunnel: w669 -> [_ _ _ w702]
                    frame #0 {
                      n274 = global write "Meas_global.vi" "Remote control"(TRUE ("Remote control")) -> ()
                    }
                    frame #1 {
                      n275 = call "Get_Data_Base_file_code.vi"("Results Filename"=w682, "Data Type"="Raw_Calibrations") -> ("Raw Data File Name"=w679:path)  [unwired: 3 out]
                      n276 = call "Measurement.vi"("setup"=Setup."Run Program", "Post Process"=Post_Process."Take New Data", "File"=Save_Data."Save No Data", "Raw data file"=w679, "Setup filename"=w678) -> ("Status Out"=w677:T2)  [unwired: 2 in, 12 out]
                    }
                    frame #2 {
                      n277 = local read "FF Indexes"() -> (w688:i16[])
                      n278 = global read "Plug_in_data_global.vi" "Equi Spaced"() -> (w687:dbl[][])
                      n279 = for {
                        tunnel: w688 -> [w694] mode=indexing
                        tunnel: [w692] -> w686 mode=indexing
                        tunnel: [w691] -> w685 mode=indexing
                        tunnel: w687 -> [w693]
                        n280 = Index Array(array=w693, index (row)=w694) -> (element=w690:dbl[])  [unwired: 1 in]
                        n281 = call "De-spiked_Stats.vi"("Raw Signal"=w690, "No of st dev to chop at"=6.0) -> ("mean"=w692:dbl, "standard deviation"=w691:dbl)  [unwired: 1 out]
                      }
                    }
                    frame #3 {
                      n282 = Greater?(x=w704, y=0.15) -> (0:w703:bool[])
                      n283 = Or Array Elements(Boolean array=w703) -> (logical OR=w697:bool)
                      n284 = Less?(x=w702, y=2) -> (x < y?=w698:bool)
                      n285 = Equal?(x=w700, y=Multi_Run_Status."Continue" ("Status Out")) -> (x = y?=w696:bool)
                      n286 = Compound Arithmetic op=AND(w696, w697, w698) -> (w695:bool)
                    }
                  }
                }
              }
              frame #2 {
                n287 = local read "FFID St Dev"() -> (w711:dbl[][])
                n288 = local read "Valve position"() -> (w715:dbl)
                n289 = local read "Concentrations"() -> (w709:dbl[])
                n290 = global read "Meas_global.vi" "Temp"() -> (w716:dbl)
                n291 = Build Array (concatenate)(w707, w706) -> (w710:dbl[])
                n292 = Build Array (concatenate)(w711, w710) -> (→"FFID St Dev":dbl[][])
                n293 = Index Array(array=w709, index=w715) -> (element=w714:dbl)
                n294 = local read "New Calib Filenames"() -> (w713:path[])
                n295 = for {
                  tunnel: w707 -> [w722] mode=indexing
                  tunnel: w716 -> [w721]
                  tunnel: w714 -> [w720]
                  tunnel: [w719] -> w708 mode=indexing
                  tunnel: w713 -> [w718] mode=indexing
                  tunnel: w706 -> [w717] mode=indexing
                  n296 = stacked-sequence {
                    tunnel: w722 -> [w728 _]
                    tunnel: w721 -> [w725 _]
                    tunnel: w720 -> [w727 _]
                    tunnel: [_ w730] -> w719
                    tunnel: w718 -> [_ w729]
                    tunnel: w717 -> [w723 _]
                    frame #0 {
                      n297 = Build Array(w727, w728, w723, 0.0 ("element"), w725) -> (w726:dbl[])
                      n298 = global write "Calib_global.vi" "Calibration Points"(w726) -> ()
                    }
                    frame #1 {
                      n299 = call "Calibration.vi"("Mode"=Calib_mode."Refit Curve", "Calib file"=w729) -> ("Coefficients"=w731:dbl[][])  [unwired: 1 in, 16 out]
                      n300 = Index Array(array=w731, index (row)=0 ("Index")) -> (element=w730:dbl[])  [unwired: 1 in]
                    }
                  }
                }
              }
            }
          }
        }
        "Coefficients" <- w644
        n301 = local write "Status"(w645) -> ()
      }
      frame "Do Another Calibration Point?" {
        n302 = local read "No of Calib Points"() -> (w747:i32)
        n303 = local read "Status"() -> (w743:T2)
        n304 = local read "Currently On"() -> (w739:i32)
        n305 = case shown="\"Terminate Run\"" w743 {
          tunnel: [w757 w758 TRUE w761] -> w745
          tunnel: [w757 w758 FALSE w761] -> w746
          frame "Continue", Default {
            w757 = TRUE
          }
          frame "Jump to Next Point" {
            w758 = TRUE
          }
          frame "Jump to Next Row" {
          }
          frame "Terminate Run" {
            w761 = FALSE
          }
        }
        n306 = Greater?(x=w747, y=w739) -> (0:w744:bool)
        n307 = Compound Arithmetic op=AND(invert "stop", w745) -> (w742:bool)
        n308 = Compound Arithmetic op=AND(w742, w746, w744) -> (w740:bool)
        n309 = case shown="False" w740 {
          tunnel: w739 -> [_ w756]
          tunnel: [w750 Auto_Calib_Case."Set Measurement Conditions" ("Currently in Case")] -> w738
          tunnel: w737 -> [w751 _]
          tunnel: w736 -> [w749 _]
          frame False {
            n310 = case shown="\"Check VI only\"" w751 {
              tunnel: [Auto_Calib_Case."End" ("Currently in Case") Auto_Calib_Case."Skip Next Frame?" ("Currently in Case")] -> w750
              tunnel: w749 -> [_ _]
              frame "Check VI only" {
              }
              frame "Run VI" {
              }
            }
          }
          frame True {
            n311 = Increment(x=w756) -> (x+1=w755:i32)
            n312 = local write "Currently On"(w755) -> ()
          }
        }
        n313 = case shown="True" "stop" {
          frame False {
          }
          frame True {
            n314 = local write "Status"(Multi_Run_Status."Terminate Run" ("Status")) -> ()
          }
        }
      }
      frame "Skip Next Frame?" {
        n315 = local read "Status"() -> (w765:T2)
        n316 = case shown="\"Tunnel Speed\", Default" w762 {
          frame "Tunnel Speed", Default {
          }
          frame "Concentration" {
            n317 = call "Fast_FID_Valve_Control.vi"("Requested Position"=4 ("Requested Posn.")) -> ()  [unwired: 7 out]
          }
        }
        n318 = case shown="\"Continue\"" w765 {
          tunnel: [w769 Auto_Calib_Case."End" ("Currently in Case")] -> w764
          tunnel: w763 -> [w769 _]
          frame "Continue" {
          }
          frame "Terminate Run", Default {
          }
        }
      }
      frame "Insert New calibration Filenames into Measurement Setup file" {
        n319 = local read "New Calib Filenames"() -> (w772:path[])
        n320 = local read "Ch No's"() -> (w782:i16[])
        n321 = global read "Meas_global.vi" "Raw data file"() -> (w779:path)
        n322 = Strip Path(path=w779) -> (stripped path=w778:path)  [unwired: 1 out]
        n323 = Equal?(x=Auto_Calib_Type."Concentration" ("Calibration varying"), y=w776) -> (x = y?=w775:bool)
        n324 = call "Current_Calib_Filenames.vi"("Calib Filename"=w772, "Channel Numbers"=w782, "Mode"=App_Global."Write to Global") -> ()  [unwired: 3 out]
        n325 = case shown="False" w775 {
          tunnel: [Auto_Calib_Case."Warn if Current Calibration fit is poor" ("Currently in Case") w788] -> w774
          tunnel: w773 -> [_ w788]
          tunnel: w772 -> [_ w787]
          tunnel: [1 w786] -> w771
          frame False {
          }
          frame True {
            n326 = Array Size(array=w787) -> (size(s)=w786:i32)
          }
        }
        n327 = for {
          N: w771 -> [_]
          tunnel: w772 -> [w790] mode=indexing
          tunnel: w778 -> [w794]
          w792 = FALSE  # Variable Target?
          n328 = Strip Path(path=w790) -> (name=w793:string)  [unwired: 1 out]
          n329 = Build Path(base path=w794, name or relative path=w793) -> (appended path=w789:path)
          n330 = call "Remember_Calib_Filenames.vi"("Filename to Remember"=w789) -> ()  [unwired: 1 out]
          n331 = call "Copy_with_Check.vi"("Mode"=enum16{"Move", "Copy"}."Copy", "Target Path"=w789, "Variable Target?"=w792, "Source Path"=w790) -> ()  [unwired: 1 out]
        }
      }
      frame "Warn if FFID calibration is very non linear" {
        w811 = FALSE  # Dialog Box (T)
        n332 = local read "Root Name"() -> (w810:string[])
        n333 = local read "Coefficients"() -> (w813:dbl[][])
        n334 = for {
          tunnel: w813 -> [w820] mode=indexing
          shift-right: [w822] -> w808
          shift-left: "" -> [w823]
          tunnel: w810 -> [w824] mode=indexing
          tunnel: [w817] -> w803 mode=indexing
          tunnel: "If the calibration fit for %s had been linear instead of a second order polynomial, it would have yielded an average fit error of %.1f%%.\\n" ("Format String") -> [w815]
          n335 = Index Array(array=w820, index=0 ("Index")) -> (element=w818:dbl)
          n336 = Absolute Value(x=w818) -> (abs(x)=w817:dbl)
          n337 = Less?(x=w817, y=2.2) -> (x < y?=w821:bool)
          n338 = case shown="False" w821 {
            tunnel: w824 -> [w826 _]
            tunnel: w817 -> [w827 _]
            tunnel: w823 -> [w830 w831]
            tunnel: [w828 w831] -> w822
            tunnel: w815 -> [w825 _]
            frame False {
              n339 = Format Into String(format string=w825, w826, w827) -> (resulting string=w829:string)  [unwired: 2 in, 1 out]
              n340 = Concatenate Strings(w830, w829) -> (w828:string)
            }
            frame True {
            }
          }
        }
        n341 = Array Max & Min(array=w803) -> (max value=w802:dbl)  [unwired: 3 out]
        n342 = Greater?(x=w802, y=7.0) -> (0:w800:bool)
        n343 = Select(t="Very Poor FFID Linearity", s=w800, f="Poor FFID Linearity") -> (s? t:f=w797:string)
        n344 = Empty String/Path?(string/path=w808) -> (empty?=w807:bool)
        n345 = Not(x=w807) -> (.not. x?=w806:bool)
        n346 = Bundle By Name(cluster=errorcluster {"status"=FALSE, "code"=0, "source"=""} ("error in (no error)"), "source"=w808, "status"=w806) -> (w805:errorcluster)
        n347 = call "EnFlo_Error_Handler.vi"("error in (no error)"=w805, "Error Type"=w797, "Dialog Box (T)"=w811) -> ()  [unwired: 3 out]
      }
      frame "Warn if FFID variance is high" {
        w853 = FALSE  # Dialog Box (T)
        n348 = local read "New Calib Filenames"() -> (w835:path[])
        n349 = local read "FFID St Dev"() -> (w855:dbl[][])
        n350 = Index Array(array=w840, index (col)=0 ("disabled index (col)")) -> (element=w838:dbl[])  [unwired: 1 in]
        n351 = Array Size(array=w835) -> (size(s)=w834:i32)
        n352 = for {
          tunnel: w855 -> [w872]
          shift-right: [w874] -> w851
          shift-left: "" -> [w875]
          tunnel: w835 -> [w863] mode=indexing
          tunnel: "For %s the measurement at %dppm had a standard deviation of %.2f volts for an average value of  %.1f volts.\\n" ("Format String") -> [w873]
          tunnel: w838 -> [w866]
          tunnel: [w865] -> w836 mode=indexing
          tunnel: w834 -> [w861]
          tunnel: [w857] -> w832 mode=indexing
          i -> [w860]
          n353 = Add(x=w861, y=w860) -> (x+y=w859:i32)
          n354 = Strip Path(path=w863) -> (name=w862:string)  [unwired: 1 out]
          n355 = Index Array(array=w872, index (col)=w860) -> (element=w864:dbl[])  [unwired: 1 in]
          n356 = Index Array(array=w872, index (col)=w859) -> (element=w858:dbl[])  [unwired: 1 in]
          n357 = Array Max & Min(array=w858) -> (min value=w857:dbl)  [unwired: 3 out]
          n358 = call <vilib>:"Mean.vi"("X"=w864) -> ("mean"=w871:dbl)  [unwired: 1 out]
          n359 = Divide(x=w858, y=w871) -> (x/y=w870:dbl[])
          n360 = Array Max & Min(array=w870) -> (max value=w865:dbl, max index (indices)=w867:i32)  [unwired: 2 out]
          n361 = Greater?(x=w865, y=0.06) -> (0:w868:bool)
          n362 = case shown="True" w868 {
            tunnel: w862 -> [_ w886]
            tunnel: w875 -> [w876 w892]
            tunnel: [w876 w890] -> w874
            tunnel: w873 -> [_ w889]
            tunnel: w867 -> [_ w887]
            tunnel: w866 -> [_ w888]
            tunnel: w865 -> [_ _]
            tunnel: w858 -> [_ w885]
            tunnel: w864 -> [_ w883]
            frame False {
            }
            frame True {
              n363 = local read "Concentrations"() -> (w881:dbl[])
              n364 = Index Array(array=w888, index=w887) -> (element=w882:dbl)
              n365 = Index Array(array=w885, index=w887) -> (element=w879:dbl)
              n366 = Index Array(array=w883, index=w887) -> (element=w884:dbl)
              n367 = Index Array(array=w881, index=w882) -> (element=w880:dbl)
              n368 = Multiply(x=w879, y=2.5) -> (x*y=w878:dbl)
              n369 = Format Into String(format string=w889, w886, w880, w878, w884) -> (resulting string=w891:string)  [unwired: 2 in, 1 out]
              n370 = Concatenate Strings(w892, w891) -> (w890:string)
            }
          }
        }
        "Minimum St Dev" <- w832
        n371 = Array Max & Min(array=w836) -> (max value=w846:dbl)  [unwired: 3 out]
        n372 = Greater?(x=w846, y=0.09) -> (0:w844:bool)
        n373 = Select(t="Very unstable FFID calibration point", s=w844, f="Unstable FFID calibration point") -> (s? t:f=w841:string)
        n374 = Empty String/Path?(string/path=w851) -> (empty?=w850:bool)
        n375 = Not(x=w850) -> (.not. x?=w849:bool)
        n376 = Bundle By Name(cluster=errorcluster {"status"=FALSE, "code"=0, "source"=""} ("error in (no error)"), "source"=w851, "status"=w849) -> (w848:errorcluster)
        n377 = call "EnFlo_Error_Handler.vi"("error in (no error)"=w848, "Error Type"=w841, "Dialog Box (T)"=w853) -> ()  [unwired: 3 out]
      }
      frame "Insert Bkgnd Variance into calib file" {
        n378 = local read "New Calib Filenames"() -> (w895:path[])
        n379 = local read "Minimum St Dev"() -> (w896:dbl[])
        n380 = local read "Coefficients"() -> (w893:dbl[][])
        n381 = for {
          tunnel: w896 -> [w901] mode=indexing
          tunnel: w895 -> [w907] mode=indexing
          tunnel: w893 -> [w904] mode=indexing
          n382 = call "Read_File_Simple.vi"("Filename"=w907) -> ("string"=w911:string)  [unwired: 2 in, 7 out]
          n383 = Index Array(array=w904, index=2) -> (element=w902:dbl)
          n384 = Multiply(x=w901, y=w902) -> (x*y=w900:dbl)
          n385 = Square(x=w900) -> (x^2=w899:dbl)
          n386 = Number To Fractional String(number=w899, precision (6)=i16 8) -> (F-format string=w909:string)  [unwired: 2 out]
          n387 = call "Replace_data_in_setup_string.vi"("New data string"=w909, "Input string"=w911, "Variable name"="Fast FID Bkgnd Variance") -> ("Appended string"=w906:string)
          n388 = call "Write_File_Simple.vi"("append to file? (new file:F)"=FALSE, "character string"=w906, "file path"=w907) -> ()  [unwired: 2 out]
        }
      }
      frame "Warn if FFID voltages are too low" {
        w929 = FALSE  # Dialog Box (T)
        n389 = local read "Coefficients"() -> (w919:dbl[][])
        n390 = local read "Concentrations"() -> (w915:dbl[])
        n391 = Index Array(array=w922, index (col)=0 ("disabled index (col)")) -> (element=w914:dbl[])  [unwired: 1 in]
        n392 = local read "New Calib Filenames"() -> (w918:path[])
        n393 = for {
          tunnel: w915 -> [w934]
          tunnel: w914 -> [w933] mode=indexing
          tunnel: [w932] -> w913 mode=indexing
          n394 = Index Array(array=w934, index=w933) -> (element=w932:dbl)
        }
        n395 = Array Max & Min(array=w913) -> (max value=w912:dbl)  [unwired: 3 out]
        n396 = for {
          shift-right: [w944] -> w927
          shift-left: "" -> [w945]
          tunnel: "For %s the maximum measured calibration voltage was %.1f volts.\nCheck that the FID is running and correctly connected to the acquisition system." ("Format String") -> [w943]
          tunnel: w919 -> [w941] mode=indexing
          tunnel: w918 -> [w937] mode=indexing
          tunnel: w912 -> [w936]
          n397 = Split 1D Array(array=w941, index=1) -> (second subarray=w940:dbl[])  [unwired: 1 out]
          n398 = call "Polybackwards.vi"("Coefficients"=w940, "Y input"=w936) -> ("X output"=w935:dbl)  [unwired: 1 out]
          n399 = Less?(x=w935, y=0.2) -> (x < y?=w938:bool)
          n400 = case shown="True" w938 {
            tunnel: w945 -> [w946 w953]
            tunnel: [w946 w951] -> w944
            tunnel: w943 -> [_ w950]
            tunnel: w937 -> [_ w949]
            tunnel: w935 -> [_ w947]
            frame False {
            }
            frame True {
              n401 = Strip Path(path=w949) -> (name=w948:string)  [unwired: 1 out]
              n402 = Format Into String(format string=w950, w948, w947) -> (resulting string=w952:string)  [unwired: 2 in, 1 out]
              n403 = Concatenate Strings(w953, w952) -> (w951:string)
            }
          }
        }
        n404 = Empty String/Path?(string/path=w927) -> (empty?=w926:bool)
        n405 = Not(x=w926) -> (.not. x?=w925:bool)
        n406 = Bundle By Name(cluster=errorcluster {"status"=FALSE, "code"=0, "source"=""} ("error in (no error)"), "source"=w927, "status"=w925) -> (w924:errorcluster)
        n407 = call "EnFlo_Error_Handler.vi"("error in (no error)"=w924, "Error Type"="Low FFID calibration voltages", "Dialog Box (T)"=w929) -> ()  [unwired: 3 out]
      }
      frame "Warn if Current Calibration fit is poor" {
        w968 = FALSE  # Dialog Box (T)
        n408 = local read "Root Name"() -> (w967:string[])
        n409 = local read "Coefficients"() -> (w970:dbl[][])
        n410 = for {
          tunnel: w970 -> [w977] mode=indexing
          shift-right: [w979] -> w965
          shift-left: "" -> [w980]
          tunnel: w967 -> [w981] mode=indexing
          tunnel: [w974] -> w960 mode=indexing
          n411 = Index Array(array=w977, index=0 ("Index")) -> (element=w975:dbl)
          n412 = Absolute Value(x=w975) -> (abs(x)=w974:dbl)
          n413 = Less?(x=w974, y=1.0) -> (x < y?=w978:bool)
          n414 = case shown="True" w978 {
            tunnel: w981 -> [w983 _]
            tunnel: w974 -> [w984 _]
            tunnel: w980 -> [w987 w988]
            tunnel: [w985 w988] -> w979
            frame False {
              n415 = Format Into String(format string="The calibration for %s has an average fit error of %.1f%%\\n" ("Format String"), w983, w984) -> (resulting string=w986:string)  [unwired: 2 in, 1 out]
              n416 = Concatenate Strings(w987, w986) -> (w985:string)
            }
            frame True {
            }
          }
        }
        n417 = Array Max & Min(array=w960) -> (max value=w959:dbl)  [unwired: 3 out]
        n418 = Greater?(x=w959, y=7.0) -> (0:w957:bool)
        n419 = Select(t="Very Poor Calibration", s=w957, f="Poor Calibration") -> (s? t:f=w954:string)
        n420 = Empty String/Path?(string/path=w965) -> (empty?=w964:bool)
        n421 = Not(x=w964) -> (.not. x?=w963:bool)
        n422 = Bundle By Name(cluster=errorcluster {"status"=FALSE, "code"=0, "source"=""} ("error in (no error)"), "source"=w965, "status"=w963) -> (w962:errorcluster)
        n423 = call "EnFlo_Error_Handler.vi"("error in (no error)"=w962, "Error Type"=w954, "Dialog Box (T)"=w968) -> ()  [unwired: 3 out]
      }
      frame "Warn if Calibration Coefficients have significantly altered" {
        w1014 = FALSE  # Dialog Box (T)
        w1001 = 8.0 ("y")
        n424 = local read "New Calib Filenames"() -> (w1006:path[])
        n425 = global read "Calib_global.vi" "Instrument type"() -> (w1004:T13)
        n426 = local read "Root Name"() -> (w1005:string[])
        n427 = Unbundle By Name(w993) -> ("Extra Commands"=w992:string)
        n428 = global read "Extra_Commands_Global.vi" "If Command"() -> (w994:string)
        n429 = call "Extra_Commands.vi"("String to Search"=w992, "Command"=w994) -> ("String Value"=w991:string)  [unwired: 1 in, 4 out]
        n430 = call "Calibration_Analysis.vi"("Root Name"=w1005, "New Calib Filenames"=w1006, "Instrument type"=w1004, "Clear Calib History"="Clear Calib History") -> ("Error String"=w1003:string, "Max % Error"=w989:dbl)
        n431 = call "Get_array_values_fr_String.vi"("String Value"=w991) -> ("Numeric Array"=w990:dbl[], "String array"=w996:string[])
        n432 = Greater?(x=w989, y=w1001) -> (0:w1002:bool)
        n433 = Index Array(array=w996, index=0 ("Index")) -> (element=w997:string)
        n434 = case shown="\"Drift Greater Than\"" w997 {
          tunnel: w990 -> [w1020 _]
          tunnel: w989 -> [w1019 _]
          frame "Drift Greater Than" {
            n435 = Index Array(array=w1020, index=1 ("Index")) -> (element=w1018:dbl)
            n436 = Greater?(x=w1019, y=w1018) -> (0:w1017:bool)
            n437 = case shown="True" w1017 {
              frame False {
              }
              frame True {
                n438 = local write "Status"(Multi_Run_Status."Jump To Fall Back" ("Status")) -> ()
              }
            }
          }
          frame "No Match", Default {
          }
        }
        n439 = Format Into String(format string="Calibration Drift Greater than %d%%", w1001) -> (resulting string=w999:string)  [unwired: 2 in, 1 out]
        n440 = Select(t=w999, s=w1002, f="Calibration Drift") -> (s? t:f=w1007:string)
        n441 = Empty String/Path?(string/path=w1003) -> (empty?=w1012:bool)
        n442 = Not(x=w1012) -> (.not. x?=w1011:bool)
        n443 = Bundle By Name(cluster=errorcluster {"status"=FALSE, "code"=0, "source"=""} ("error in (no error)"), "source"=w1003, "status"=w1011) -> (w1010:errorcluster)
        n444 = call "EnFlo_Error_Handler.vi"("error in (no error)"=w1010, "Error Type"=w1007, "Dialog Box (T)"=w1014) -> ()  [unwired: 3 out]
      }
      frame "End" {
        n445 = local read "Original Calib File"() -> (w1027:path)
        n446 = Bundle By Name(cluster=w1024, "Filename"=w1027) -> ()  [unwired: 1 out]
        n447 = case shown="\"Concentration\"" w1026 {
          tunnel: w1024 -> [_ w1043]
          tunnel: w1025 -> [_ w1031]
          tunnel: w1023 -> [_ w1042]
          frame "Tunnel Speed", Default {
          }
          frame "Concentration" {
            n448 = Unbundle By Name(w1043) -> ("Averaging time (min)"=w1045:dbl)
            n449 = global read "Trav_pos_global.vi" "Simulation Time"() -> (w1034:timestamp)
            n450 = Unbundle By Name(w1043) -> ("Start X"=w1051:dbl, "Start Y"=w1050:dbl, "Start Z"=w1049:dbl)
            n451 = Build Array(w1051, w1050, w1049) -> (w1052:dbl[])
            n452 = Select(t=3 ("No. of pts."), s=w1042, f=2 ("No. of pts.")) -> (s? t:f=w1036:i32)
            n453 = call "Coordinate_Trans_.vi"("Input Position"=w1052) -> ("X"=w1048:dbl, "Y"=w1047:dbl, "Z"=w1046:dbl)
            n454 = Multiply(x=60.0, y=w1045) -> (x*y=w1039:dbl)
            n455 = Add(x=w1046, y=50.0) -> (x+y=w1053:dbl)
            n456 = Add(x=w1039, y=60.0) -> (x+y=w1037:dbl)
            n457 = Bundle By Name(cluster=w1043, "Start X"=w1048, "Start Y"=w1047, "Start Z"=w1053) -> (w1054:T5)
            n458 = Multiply(x=w1037, y=w1036) -> (x*y=w1035:dbl)
            n459 = Add(x=w1034, y=w1035) -> (x+y=w1032:timestamp)
            n460 = call "Set_Traverse_Position.vi"("Simulate/Run"=w1031, "Currently on Point"=1, "Traverse line"=w1054) -> ()  [unwired: 3 out]
            n461 = call "Run_FFID_Bkgnd.vi"("Simulated Time"=w1032, "Run Now?"=TRUE, "Simulate/Run"=w1031) -> ()  [unwired: 3 out]
          }
        }
        "Traverse Out" <- w1024
      }
    }
    "Currently in Case" <- w8
  }
  "Error Messages" <- w3
